vi "swerve_output_scaling.vi"(8 "d":dbl, 9 "c":dbl, 10 "b":dbl, 11 "a":dbl) -> (0 "d scaled":dbl, 1 "c scaled":dbl, 2 "b scaled":dbl, 3 "a scaled":dbl)   [LabVIEW 2020]
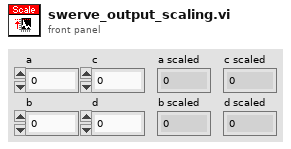
[diagram p1: front panel]
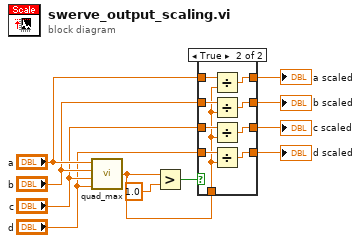
[diagram p0: block diagram]
diagram:
  n1 = call "quad_max.vi"("d"="d", "c"="c", "b"="b", "a"="a") -> ("max"=w1:dbl)
  n2 = Greater?(x=w1, y=1.0) -> (0:w6:bool)
  n3 = case shown="True" w6 {
    tunnel: "a" -> [w15 w24]
    tunnel: "b" -> [w14 w23]
    tunnel: "c" -> [w13 w22]
    tunnel: "d" -> [w12 w21]
    tunnel: [w12 w20] -> w5
    tunnel: [w13 w19] -> w4
    tunnel: [w14 w18] -> w2
    tunnel: [w15 w17] -> w3
    tunnel: w1 -> [_ w16]
    frame False {
    }
    frame True {
      n4 = Divide(x=w24, y=w16) -> (x/y=w17:dbl)
      n5 = Divide(x=w23, y=w16) -> (x/y=w18:dbl)
      n6 = Divide(x=w22, y=w16) -> (x/y=w19:dbl)
      n7 = Divide(x=w21, y=w16) -> (x/y=w20:dbl)
    }
  }
  "a scaled" <- w3
  "b scaled" <- w2
  "c scaled" <- w4
  "d scaled" <- w5
